vi "TDMSViewerRunningFlag.vi"(0 "RunningIn":bool, 7 "Write":bool, 11 "error in":errorcluster) -> (4 "RunningOut":bool, 15 "error out":errorcluster)   [LabVIEW 2025, in "ZE_Recorder.lvlib"]
doc: "ZE_Recorder.lvlib:TDMSViewerRunningFlag.vi\n----------------------------------------------\nStorage VI for a Boolean. This VI is used to store, if the TDMS Viewer is running or not\n\nInputs:\n---------------------\n- : Cluster; \n- : Boolean; \n- : Boolean; \n\nOutputs:\n---------------------\n- : Cluster; \n- : Boolean; \n\n----------------------------------------------\n13.08.2020, wer\nZühlke Engineering AG\nCH-8952 Schlieren\nwww.zuehlke.com"
uses:
  ZE_Recorder.lvlib
panel:
  # "Connector Pane"
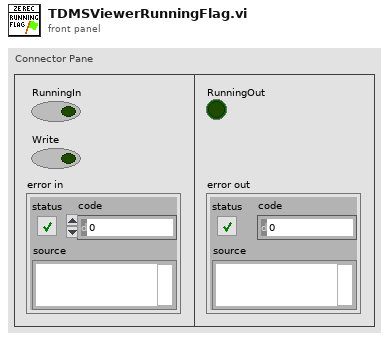
[diagram p1: front panel]
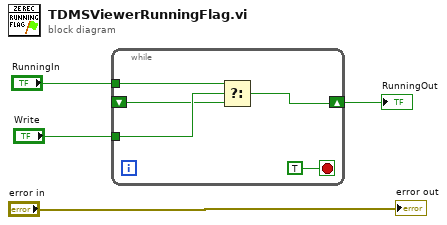
[diagram p0: block diagram]
diagram:
  n1 = while {
    shift-right: [w6] -> w1
    shift-left: _ -> [w7]
    tunnel: "Write" -> [w9]
    tunnel: "RunningIn" -> [w8]
    stop <- TRUE stop-if-true
    n2 = Select(t=w8, s=w9, f=w7) -> (s? t:f=w6:bool)
  }
  "RunningOut" <- w1
  "error out" <- "error in"
